vi "convert unix time to lv timestamp.vi"(11 "UNIX Time (seconds)":dbl) -> (3 "LV Time Stamp":timestamp)   [LabVIEW 2013, in "Linux RT Utilities.lvlib"]
uses:
  Linux RT Utilities.lvlib
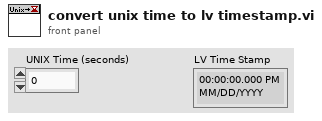
[diagram p1: front panel]
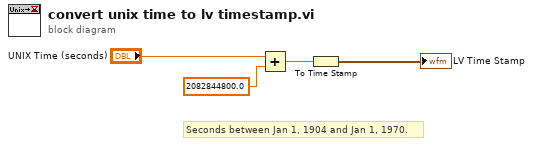
[diagram p0: block diagram]
diagram:
  # "Seconds between Jan 1, 1904 and Jan 1, 1970."
  n1 = Add(x="UNIX Time (seconds)", y=2082844800.0) -> (x+y=w2:dbl)
  n2 = To Time Stamp(1:w2) -> (0:→"LV Time Stamp":timestamp)
